vi "Apply Theme.vi"(8 "Error In":errorcluster, 10 "Override Root With (Empty)":string, 11 "Appearance Actor in":refnum<class "Appearance Actor.lvclass">) -> (0 "Error Out":errorcluster, 3 "Appearance Actor out":refnum<class "Appearance Actor.lvclass">)   [LabVIEW 2021, in "Appearance Actor.lvlib" / "Appearance Actor.lvclass"]
doc: "Apply the loaded theme to the current Actor.\n\nBy default, needs UI Control References to be listed in <B>Appearance Actor</B> internal data. But you can override this vi to do it your own way."
uses:
  Appearance Actor.lvclass
  Appearance Actor.lvclass/Appearance Actor.ctl
  Theme Classes/Generic Theme/API/Typedefs/Window Element--enum.ctl
  Theme Classes/Generic Theme/Generic Theme.lvclass
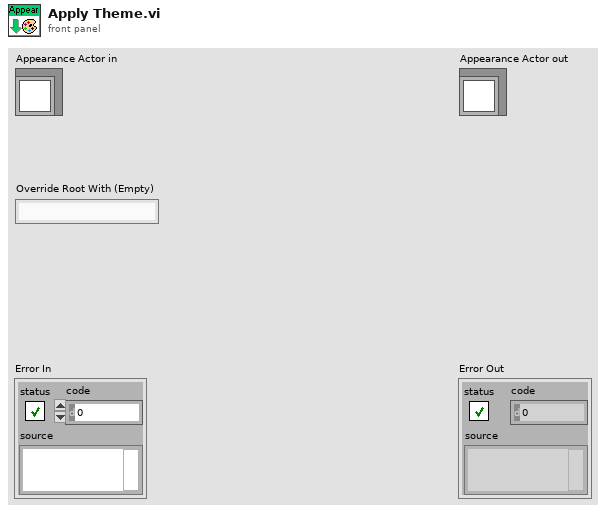
[diagram p1: front panel]
types:
  T1 = typedef "Appearance Actor.lvlib/Generic Theme.lvclass/Window Element--enum.ctl" = enum16{"None", "TB", "SM", "BP", "SB"}
  T2 = typedef "Appearance Actor.lvlib/Appearance Actor.lvclass/Control Reference Lists--cluster.ctl" = cluster{"TitleBar":T3, "SideMenu":T4, "BodyPane":T5, "StatusBar":T6}
  T3 = typedef "Appearance Actor.lvlib/Appearance Actor.lvclass/Control Reference Lists-TitleBar--cluster.ctl" = cluster{"Pane":refnum<vi>[], "Title":refnum<vi>, "Dark-CloseButton":refnum<vi>, "Light-CloseButton":refnum<vi>, "Dark-Buttons":refnum<vi>[], "Light-Buttons":refnum<vi>[], "Splitter":refnum<vi>}
  T4 = typedef "Appearance Actor.lvlib/Appearance Actor.lvclass/Control Reference Lists-SideMenu--cluster.ctl" = cluster{"Pane":refnum<vi>[], "Dark-Buttons":refnum<vi>[], "Light-Buttons":refnum<vi>[], "Splitter":refnum<vi>}
  T5 = typedef "Appearance Actor.lvlib/Appearance Actor.lvclass/Control Reference Lists-BodyPane--cluster.ctl" = cluster{"Pane":refnum<vi>[]}
  T6 = typedef "Appearance Actor.lvlib/Appearance Actor.lvclass/Control Reference Lists-StatusBar--cluster.ctl" = cluster{"Pane":refnum<vi>[], "Dark-Buttons":refnum<vi>[], "Light-Buttons":refnum<vi>[], "Splitter":refnum<vi>}
  T7 = typedef "Appearance Actor.lvlib/Generic Theme.lvclass/Theme Info--cluster.ctl" = cluster{"Name":string, "Type":string, "Version":string}
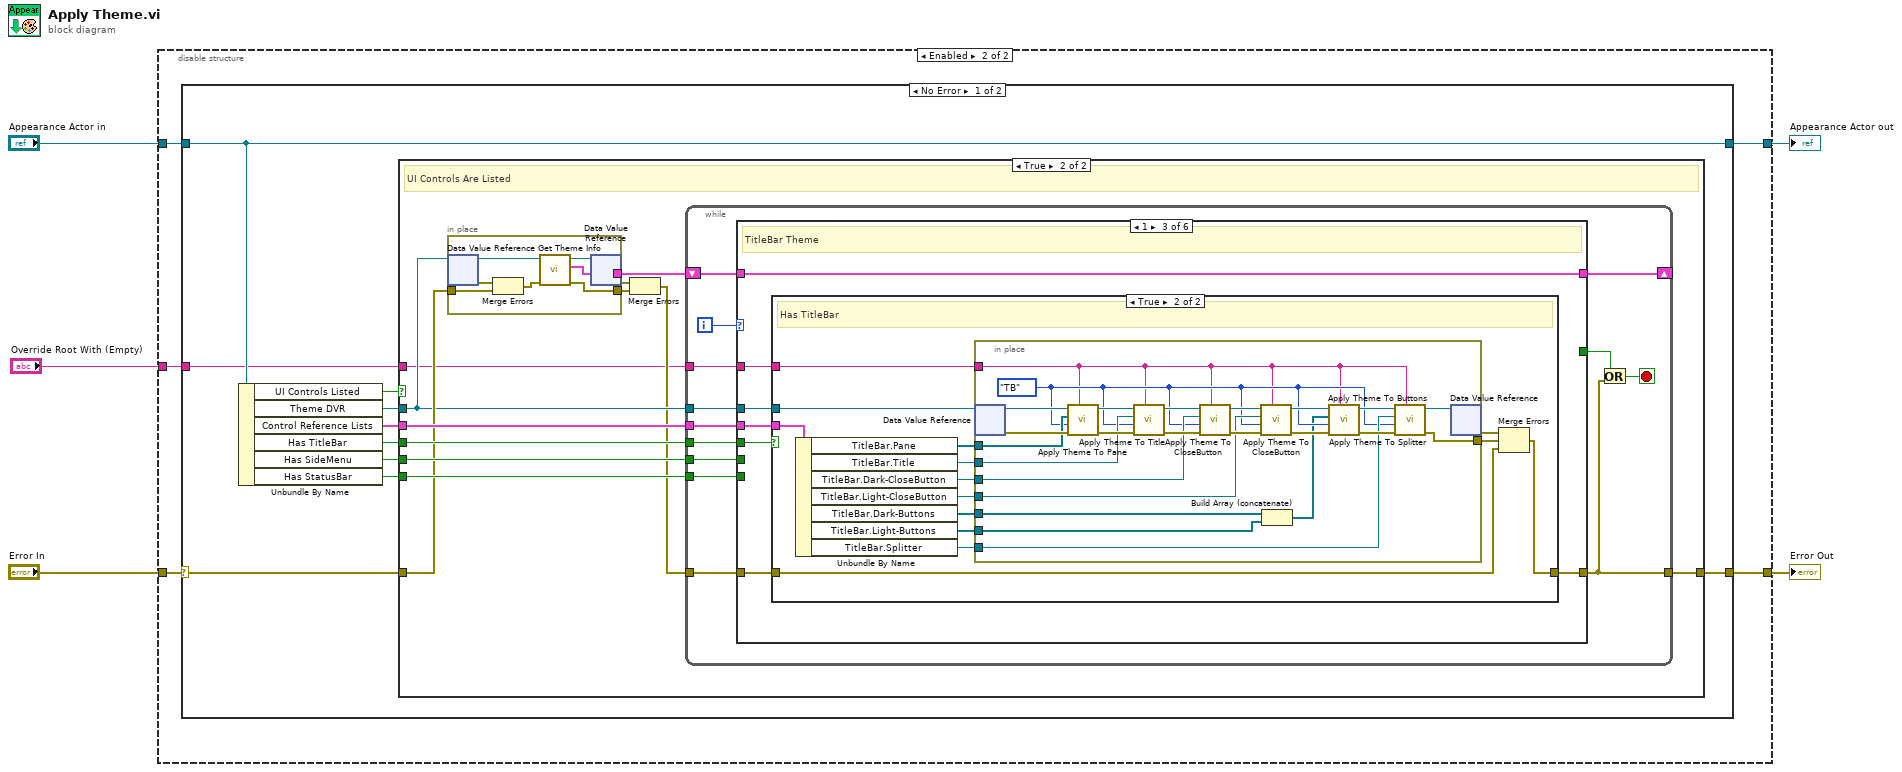
[diagram p0: block diagram]
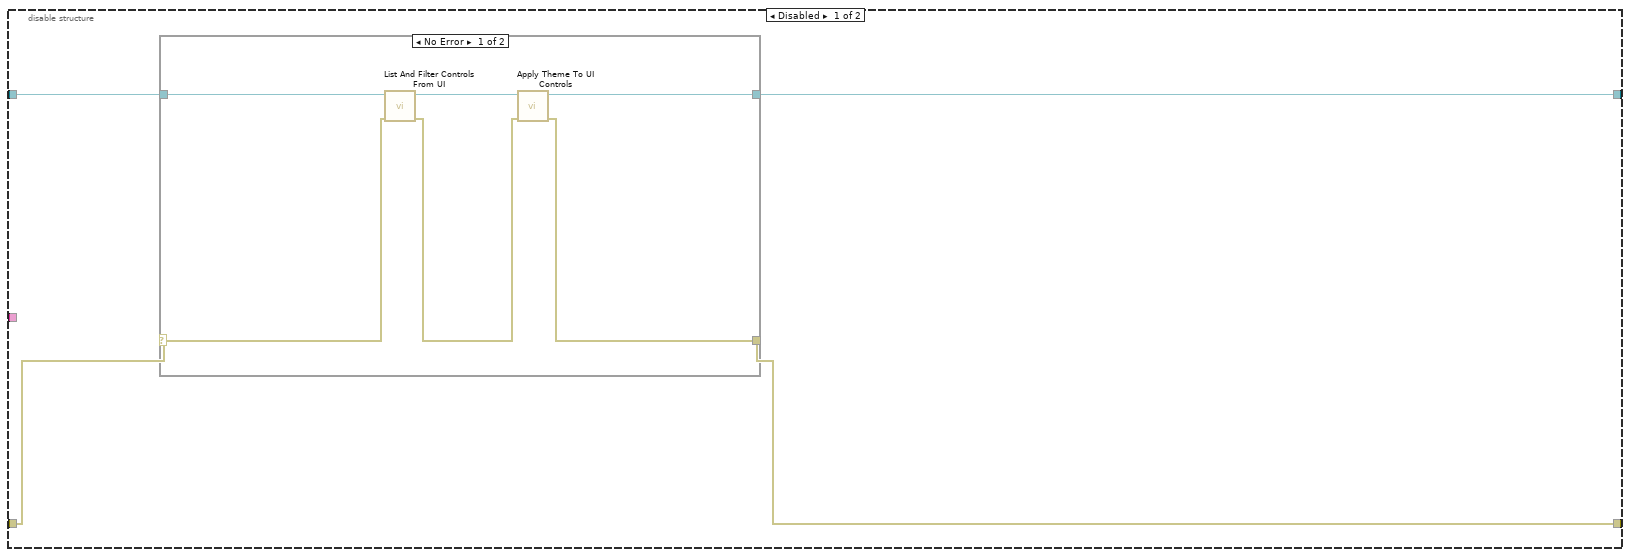
[diagram p2: hidden frame]
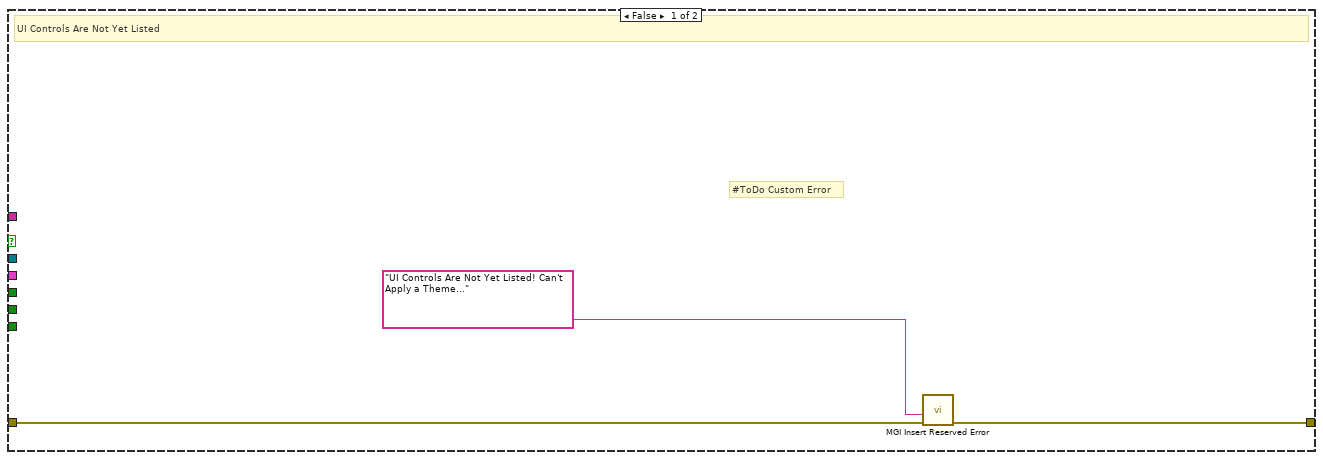
[diagram p4: hidden frame]
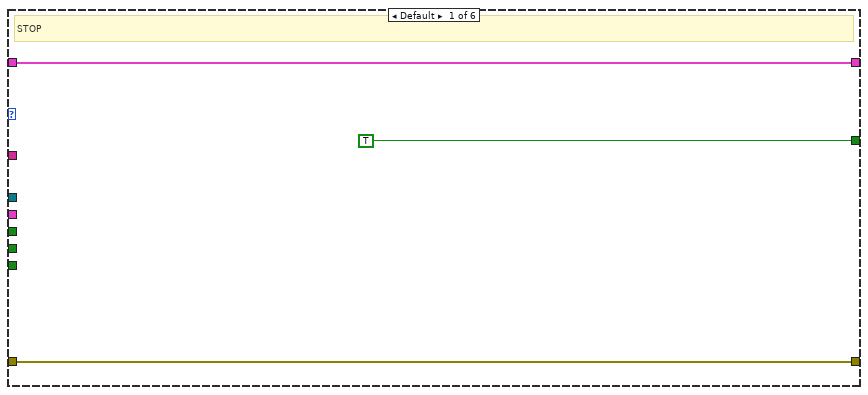
[diagram p5: hidden frame]
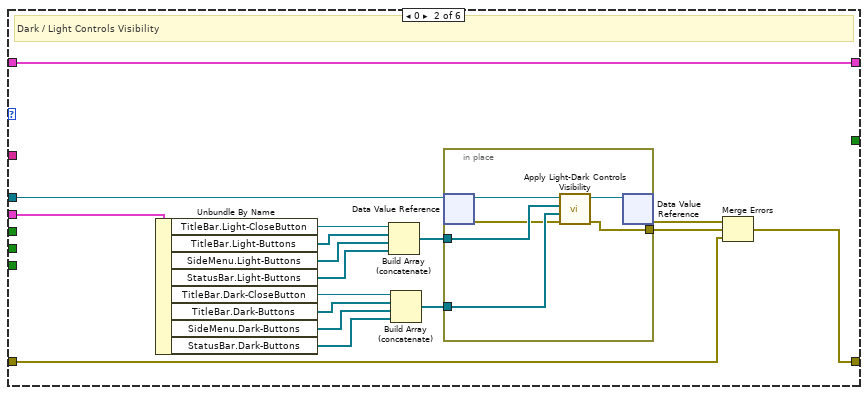
[diagram p6: hidden frame]
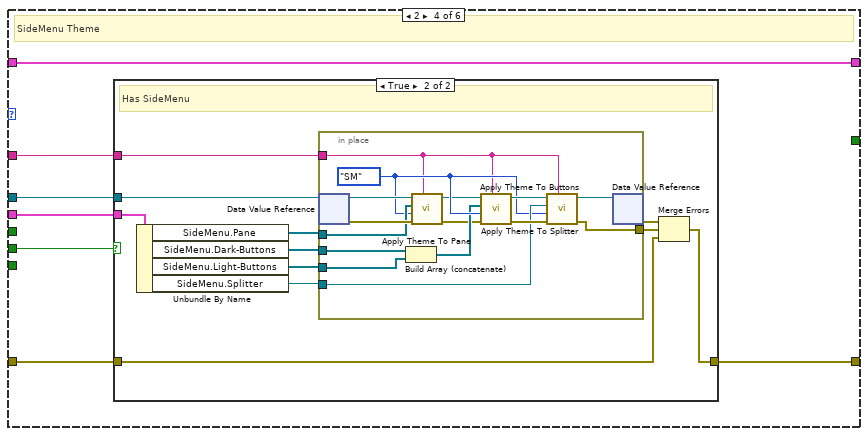
[diagram p8: hidden frame]
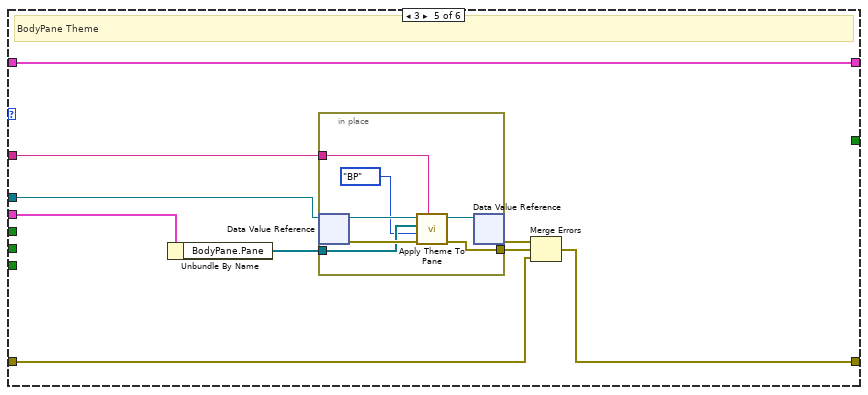
[diagram p10: hidden frame]
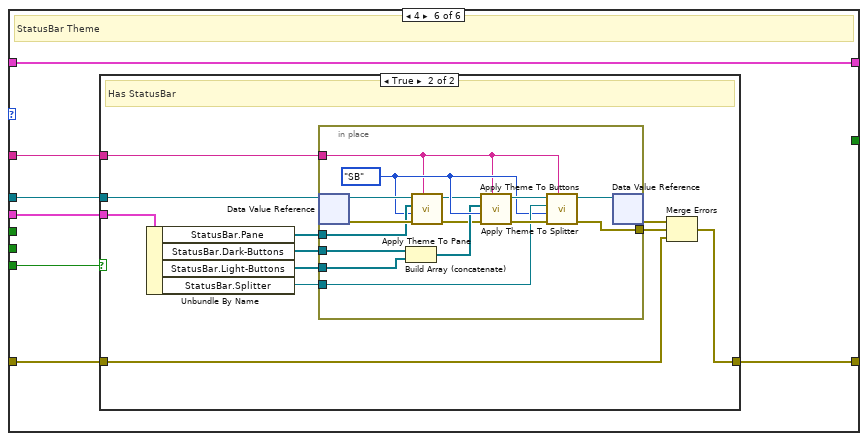
[diagram p11: hidden frame]
diagram:
  n1 = disable-structure shown="Enabled" {
    disable-tunnel: "Error In" -> [w9 w21]
    disable-tunnel: [w8 w19] -> w4
    disable-tunnel: "Appearance Actor in" -> [w7 w22]
    disable-tunnel: [w6 w20] -> w2
    disable-tunnel: "Override Root With (Empty)" -> [_ w18]
    frame Disabled {
      n2 = case shown="No Error" w9 {
        selector: w9 -> [w13 w17]
        tunnel: [w11 w17] -> w8
        tunnel: [w14 w16] -> w6
        tunnel: w7 -> [w10 w16]
        frame No Error {
          n3 = call "List And Filter Controls From UI.vi"("Error In"=w13, "Appearance Actor In"=w10) -> ("Error Out"=w12:errorcluster, "Appearance Actor Out"=w15:refnum<class "Appearance Actor.lvclass">)  [unwired: 8 in]
          n4 = call "Apply Theme To UI Controls.vi"("Error In"=w12, "Appearance Actor in"=w15) -> ("Error Out"=w11:errorcluster, "Appearance Actor out"=w14:refnum<class "Appearance Actor.lvclass">)  [unwired: 8 in]
        }
        frame Error {
        }
      }
    }
    frame Enabled {
      n5 = case shown="No Error" w21 {
        selector: w21 -> [w30 w225]
        tunnel: [w29 w225] -> w19
        tunnel: [w32 w224] -> w20
        tunnel: w22 -> [w32 w224]
        tunnel: w18 -> [w23 _]
        frame No Error {
          n6 = Unbundle By Name(w32) -> ("UI Controls Listed"=w24:bool, "Theme DVR"=w31:refnum<data-value>, "Control Reference Lists"=w28:T2, "Has TitleBar"=w27:bool, "Has SideMenu"=w26:bool, "Has StatusBar"=w25:bool)
          n7 = case shown="True" w24 {
            tunnel: w31 -> [_ w40]
            tunnel: w30 -> [w35 w41]
            tunnel: [w34 w47] -> w29
            tunnel: w28 -> [_ w46]
            tunnel: w27 -> [_ w45]
            tunnel: w26 -> [_ w44]
            tunnel: w25 -> [_ w43]
            tunnel: w23 -> [_ w36]
            frame False {
              # "#ToDo Custom Error"
              # "UI Controls Are Not Yet Listed"
              n8 = call <userlib>:"MGI Insert Reserved Error.vi"("Error In"=w35, "Error Description"="UI Controls Are Not Yet Listed! Can't Apply a Theme..." ("format string")) -> ("Error Out"=w34:errorcluster)  [unwired: 9 in]
            }
            frame True {
              # "UI Controls Are Listed"
              n9 = in-place {
                in-place-border: [w54] -> w42
                in-place-border: w41 -> [w48]
                in-place-border: [w53] -> w37
                n10 = in-place-dvr #1(w40) -> (w52:refnum<class "Generic Theme.lvclass">, w50:errorcluster)
                n11 = Merge Errors(w50, w48) -> (w49:errorcluster)
                n12 = call-dynamic "Get Theme Info.vi"("Error In"=w49, "Generic Theme in"=w52) -> ("Error Out"=w53:errorcluster, "Theme Info"=w54:T7, "Generic Theme out"=w51:refnum<class "Generic Theme.lvclass">)  [unwired: 7 in]
                n13 = in-place-dvr #1(w51) -> (w38:errorcluster)  [unwired: 1 out]
              }
              n14 = Merge Errors(w38, w37) -> (w39:errorcluster)
              n15 = while {
                tunnel: w40 -> [w66]
                tunnel: w46 -> [w65]
                tunnel: w39 -> [w61]
                tunnel: [w62] -> w47
                tunnel: w45 -> [w60]
                tunnel: w44 -> [w59]
                tunnel: w43 -> [w58]
                shift-right: [w57] -> _
                shift-left: w42 -> [w56]
                tunnel: w36 -> [w55]
                i -> [w67]
                stop <- w63 stop-if-true
                n16 = case shown="1" w67 {
                  tunnel: w66 -> [_ w73 w100 w146 w182 w196]
                  tunnel: w65 -> [_ w84 w98 w143 w179 w194]
                  tunnel: [TRUE _ _ _ _ _] -> w64
                  tunnel: w61 -> [w69 w74 w96 w142 w176 w192]
                  tunnel: [w69 w85 w99 w145 w180 w195] -> w62
                  tunnel: w60 -> [_ _ w97 _ _ _]
                  tunnel: w59 -> [_ _ _ w144 _ _]
                  tunnel: w58 -> [_ _ _ _ _ w193]
                  tunnel: [w68 w72 w95 w141 w175 w191] -> w57
                  tunnel: w56 -> [w68 w72 w95 w141 w175 w191]
                  tunnel: w55 -> [_ _ w94 w140 w174 w190]
                  frame Default {
                    # "STOP"
                  }
                  frame 0 {
                    # "Dark / Light Controls Visibility"
                    n17 = Unbundle By Name(w84) -> ("TitleBar.Light-CloseButton"=w83:refnum<vi>, "TitleBar.Light-Buttons"=w82:refnum<vi>[], "SideMenu.Light-Buttons"=w81:refnum<vi>[], "StatusBar.Light-Buttons"=w80:refnum<vi>[], "TitleBar.Dark-CloseButton"=w79:refnum<vi>, "TitleBar.Dark-Buttons"=w78:refnum<vi>[], "SideMenu.Dark-Buttons"=w77:refnum<vi>[], "StatusBar.Dark-Buttons"=w76:refnum<vi>[])
                    n18 = Build Array (concatenate)(w83, w82, w81, w80) -> (w71:refnum<vi>[])
                    n19 = Build Array (concatenate)(w79, w78, w77, w76) -> (w75:refnum<vi>[])
                    n20 = in-place {
                      in-place-border: [w92] -> w86
                      in-place-border: w71 -> [w91]
                      in-place-border: w75 -> [w90]
                      n21 = in-place-dvr #2(w73) -> (w89:refnum<class "Generic Theme.lvclass">, w88:errorcluster)
                      n22 = call-dynamic "Apply Light-Dark Controls Visibility.vi"("Error In"=w88, "Dark Controls"=w90, "Light Controls"=w91, "Generic Theme in"=w89) -> ("Error Out"=w92:errorcluster, "Generic Theme out"=w93:refnum<class "Generic Theme.lvclass">)  [unwired: 6 in]
                      n23 = in-place-dvr #2(w93) -> (w87:errorcluster)  [unwired: 1 out]
                    }
                    n24 = Merge Errors(w87, w86, w74) -> (w85:errorcluster)
                  }
                  frame 1 {
                    # "TitleBar Theme"
                    n25 = case shown="True" w97 {
                      tunnel: w100 -> [_ w115]
                      tunnel: [w101 w112] -> w99
                      tunnel: w98 -> [_ w111]
                      tunnel: w96 -> [w101 w103]
                      tunnel: w94 -> [_ w102]
                      frame False {
                        # "No TitleBar"
                      }
                      frame True {
                        # "Has TitleBar"
                        n26 = Unbundle By Name(w111) -> ("TitleBar.Pane"=w110:refnum<vi>[], "TitleBar.Title"=w109:refnum<vi>, "TitleBar.Dark-CloseButton"=w108:refnum<vi>, "TitleBar.Light-CloseButton"=w105:refnum<vi>, "TitleBar.Dark-Buttons"=w107:refnum<vi>[], "TitleBar.Light-Buttons"=w104:refnum<vi>[], "TitleBar.Splitter"=w106:refnum<vi>)
                        n27 = in-place {
                          in-place-border: [w131] -> w113
                          in-place-border: w110 -> [w129]
                          in-place-border: w109 -> [w128]
                          in-place-border: w108 -> [w127]
                          in-place-border: w107 -> [w119]
                          in-place-border: w106 -> [w126]
                          in-place-border: w105 -> [w121]
                          in-place-border: w104 -> [w118]
                          in-place-border: w102 -> [w116]
                          w120 = Window_Element--enum."TB" ("Window Element")
                          n28 = in-place-dvr #3(w115) -> (w139:refnum<class "Generic Theme.lvclass">, w138:errorcluster)
                          n29 = call-dynamic "Apply Theme To Pane.vi"("Override Root With (Empty)"=w116, "Error In"=w138, "Window Element"=w120, "Pane Refs"=w129, "Generic Theme in"=w139) -> ("Error Out"=w134:errorcluster, "Generic Theme out"=w137:refnum<class "Generic Theme.lvclass">)  [unwired: 5 in]
                          n30 = call-dynamic "Apply Theme To Title.vi"("Override Root With (Empty)"=w116, "Error In"=w134, "Window Element"=w120, "Title Ref"=w128, "Generic Theme in"=w137) -> ("Error Out"=w133:errorcluster, "Generic Theme out"=w136:refnum<class "Generic Theme.lvclass">)  [unwired: 5 in]
                          n31 = call-dynamic "Apply Theme To CloseButton.vi"("Override Root With (Empty)"=w116, "Error In"=w133, "Window Element"=w120, "CloseButton Ref"=w127, "Generic Theme in"=w136) -> ("Error Out"=w125:errorcluster, "Generic Theme out"=w124:refnum<class "Generic Theme.lvclass">)  [unwired: 5 in]
                          n32 = call-dynamic "Apply Theme To CloseButton.vi"("Override Root With (Empty)"=w116, "Error In"=w125, "Window Element"=w120, "CloseButton Ref"=w121, "Generic Theme in"=w124) -> ("Error Out"=w122:errorcluster, "Generic Theme out"=w123:refnum<class "Generic Theme.lvclass">)  [unwired: 5 in]
                          n33 = Build Array (concatenate)(w119, w118) -> (w117:refnum<vi>[])
                          n34 = call-dynamic "Apply Theme To Buttons.vi"("Override Root With (Empty)"=w116, "Error In"=w122, "Window Element"=w120, "Buttons Ref"=w117, "Generic Theme in"=w123) -> ("Error Out"=w132:errorcluster, "Generic Theme out"=w135:refnum<class "Generic Theme.lvclass">)  [unwired: 5 in]
                          n35 = call-dynamic "Apply Theme To Splitter.vi"("Override Root With (Empty)"=w116, "Error In"=w132, "Window Element"=w120, "Splitter Ref"=w126, "Generic Theme in"=w135) -> ("Error Out"=w131:errorcluster, "Generic Theme out"=w130:refnum<class "Generic Theme.lvclass">)  [unwired: 5 in]
                          n36 = in-place-dvr #3(w130) -> (w114:errorcluster)  [unwired: 1 out]
                        }
                        n37 = Merge Errors(w114, w113, w103) -> (w112:errorcluster)
                      }
                    }
                  }
                  frame 2 {
                    # "SideMenu Theme"
                    n38 = case shown="True" w144 {
                      tunnel: w146 -> [_ w158]
                      tunnel: [w147 w155] -> w145
                      tunnel: w143 -> [_ w154]
                      tunnel: w142 -> [w147 w149]
                      tunnel: w140 -> [_ w148]
                      frame False {
                        # "No SideMenu"
                      }
                      frame True {
                        # "Has SideMenu"
                        n39 = Unbundle By Name(w154) -> ("SideMenu.Pane"=w153:refnum<vi>[], "SideMenu.Dark-Buttons"=w152:refnum<vi>[], "SideMenu.Light-Buttons"=w151:refnum<vi>[], "SideMenu.Splitter"=w150:refnum<vi>)
                        n40 = in-place {
                          in-place-border: [w160] -> w156
                          in-place-border: w153 -> [w168]
                          in-place-border: w152 -> [w165]
                          in-place-border: w150 -> [w167]
                          in-place-border: w151 -> [w164]
                          in-place-border: w148 -> [w159]
                          w166 = Window_Element--enum."SM" ("Window Element")
                          n41 = in-place-dvr #4(w158) -> (w173:refnum<class "Generic Theme.lvclass">, w172:errorcluster)
                          n42 = Build Array (concatenate)(w165, w164) -> (w163:refnum<vi>[])
                          n43 = call-dynamic "Apply Theme To Pane.vi"("Override Root With (Empty)"=w159, "Error In"=w172, "Window Element"=w166, "Pane Refs"=w168, "Generic Theme in"=w173) -> ("Error Out"=w161:errorcluster, "Generic Theme out"=w162:refnum<class "Generic Theme.lvclass">)  [unwired: 5 in]
                          n44 = call-dynamic "Apply Theme To Buttons.vi"("Override Root With (Empty)"=w159, "Error In"=w161, "Window Element"=w166, "Buttons Ref"=w163, "Generic Theme in"=w162) -> ("Error Out"=w170:errorcluster, "Generic Theme out"=w171:refnum<class "Generic Theme.lvclass">)  [unwired: 5 in]
                          n45 = call-dynamic "Apply Theme To Splitter.vi"("Override Root With (Empty)"=w159, "Error In"=w170, "Window Element"=w166, "Splitter Ref"=w167, "Generic Theme in"=w171) -> ("Error Out"=w160:errorcluster, "Generic Theme out"=w169:refnum<class "Generic Theme.lvclass">)  [unwired: 5 in]
                          n46 = in-place-dvr #4(w169) -> (w157:errorcluster)  [unwired: 1 out]
                        }
                        n47 = Merge Errors(w157, w156, w149) -> (w155:errorcluster)
                      }
                    }
                  }
                  frame 3 {
                    # "BodyPane Theme"
                    n48 = Unbundle By Name(w179) -> ("BodyPane.Pane"=w178:refnum<vi>[])
                    n49 = in-place {
                      in-place-border: w178 -> [w187]
                      in-place-border: [w184] -> w177
                      in-place-border: w174 -> [w183]
                      n50 = in-place-dvr #5(w182) -> (w189:refnum<class "Generic Theme.lvclass">, w188:errorcluster)
                      n51 = call-dynamic "Apply Theme To Pane.vi"("Override Root With (Empty)"=w183, "Error In"=w188, "Window Element"=Window_Element--enum."BP", "Pane Refs"=w187, "Generic Theme in"=w189) -> ("Error Out"=w184:errorcluster, "Generic Theme out"=w185:refnum<class "Generic Theme.lvclass">)  [unwired: 5 in]
                      n52 = in-place-dvr #5(w185) -> (w181:errorcluster)  [unwired: 1 out]
                    }
                    n53 = Merge Errors(w181, w177, w176) -> (w180:errorcluster)
                  }
                  frame 4 {
                    # "StatusBar Theme"
                    n54 = case shown="True" w193 {
                      tunnel: w196 -> [_ w208]
                      tunnel: [w197 w206] -> w195
                      tunnel: w194 -> [_ w205]
                      tunnel: w192 -> [w197 w199]
                      tunnel: w190 -> [_ w198]
                      frame False {
                        # "No StatusBar"
                      }
                      frame True {
                        # "Has StatusBar"
                        n55 = Unbundle By Name(w205) -> ("StatusBar.Pane"=w204:refnum<vi>[], "StatusBar.Dark-Buttons"=w203:refnum<vi>[], "StatusBar.Light-Buttons"=w201:refnum<vi>[], "StatusBar.Splitter"=w202:refnum<vi>)
                        n56 = in-place {
                          in-place-border: w204 -> [w218]
                          in-place-border: w203 -> [w215]
                          in-place-border: w202 -> [w217]
                          in-place-border: w201 -> [w214]
                          in-place-border: [w210] -> w200
                          in-place-border: w198 -> [w209]
                          w216 = Window_Element--enum."SB" ("Window Element")
                          n57 = in-place-dvr #6(w208) -> (w223:refnum<class "Generic Theme.lvclass">, w222:errorcluster)
                          n58 = Build Array (concatenate)(w215, w214) -> (w213:refnum<vi>[])
                          n59 = call-dynamic "Apply Theme To Pane.vi"("Override Root With (Empty)"=w209, "Error In"=w222, "Window Element"=w216, "Pane Refs"=w218, "Generic Theme in"=w223) -> ("Error Out"=w211:errorcluster, "Generic Theme out"=w212:refnum<class "Generic Theme.lvclass">)  [unwired: 5 in]
                          n60 = call-dynamic "Apply Theme To Buttons.vi"("Override Root With (Empty)"=w209, "Error In"=w211, "Window Element"=w216, "Buttons Ref"=w213, "Generic Theme in"=w212) -> ("Error Out"=w220:errorcluster, "Generic Theme out"=w221:refnum<class "Generic Theme.lvclass">)  [unwired: 5 in]
                          n61 = call-dynamic "Apply Theme To Splitter.vi"("Override Root With (Empty)"=w209, "Error In"=w220, "Window Element"=w216, "Splitter Ref"=w217, "Generic Theme in"=w221) -> ("Error Out"=w210:errorcluster, "Generic Theme out"=w219:refnum<class "Generic Theme.lvclass">)  [unwired: 5 in]
                          n62 = in-place-dvr #6(w219) -> (w207:errorcluster)  [unwired: 1 out]
                        }
                        n63 = Merge Errors(w207, w200, w199) -> (w206:errorcluster)
                      }
                    }
                  }
                }
                n64 = Or(x=w64, y=w62) -> (x .or. y?=w63:bool)
              }
            }
          }
        }
        frame Error {
        }
      }
    }
  }
  "Error Out" <- w4
  "Appearance Actor out" <- w2
